vi "DHE_binning.vi"(0 "fd":i32, 5 "xbin":u8=1 min=1 max=8 step=1, 7 "ybin":u8=1 min=1 max=8 step=1, 11 "error in (no error)":errorcluster) -> (4 "fd out":i32, 8 "return value":i32, 15 "error out":errorcluster)   [LabVIEW 2016]
doc: "This VI closes the I/O interface with the instrument."
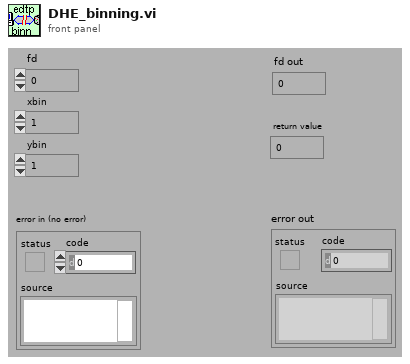
[diagram p1: front panel]
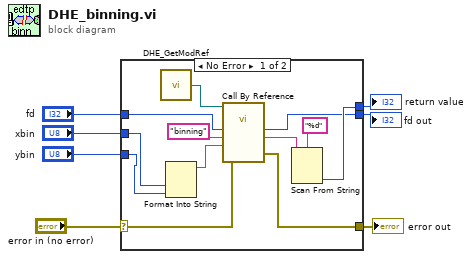
[diagram p0: block diagram]
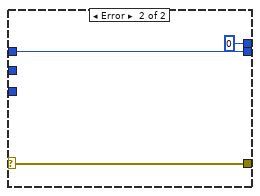
[diagram p2: hidden frame]
diagram:
  n1 = case shown="No Error" "error in (no error)" {
    selector: "error in (no error)" -> [w14 w20]
    tunnel: "fd" -> [w10 w22]
    tunnel: [w12 0] -> w6
    tunnel: [w13 w20] -> w5
    tunnel: "xbin" -> [w9 _]
    tunnel: "ybin" -> [w8 _]
    tunnel: [w11 w22] -> w2
    frame No Error {
      n2 = call "DHE_GetModRef.vi"() -> ("DHE_ModRef"=w19:refnum<vi>)  [unwired: 9 out]
      n3 = Format Into String(w9, w8) -> (resulting string=w15:string)  [unwired: 3 in, 1 out]
      n4 = call-by-ref "?"(reference=w19, "error in (no error)"=w14, "arguments"=w15, "function"="binning", "fd in"=w10) -> ("error out"=w13:errorcluster, "str result"=w17:string, "fd out"=w11:i32)  [unwired: 5 in, 3 out]
      n5 = Scan From String(format string="%d", input string=w17) -> (output 1=w12:i32)  [unwired: 2 in, 4 out]
    }
    frame Error {
    }
  }
  "error out" <- w5
  "return value" <- w6
  "fd out" <- w2
